vi "sub-Language buffer.vi"(7 "operation":enum16{"clear", "add", "get"}(ring), 10 "str":string, 11 "ID":u32 format="%04x") -> (2 "str out":string, 3 "ID out":u32)   [LabVIEW 2011]
panel:
  out "allid":u32[](array[numeric]) format="%04x"
  out "all":string[](array[string])
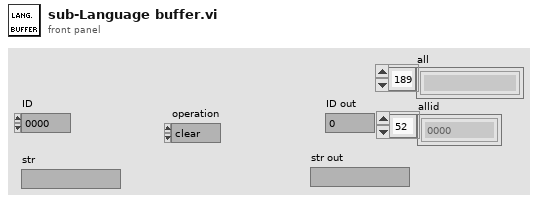
[diagram p1: front panel]
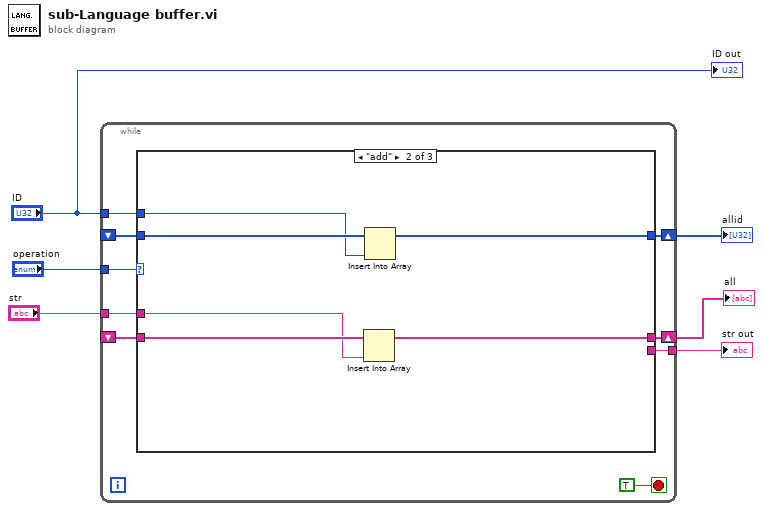
[diagram p0: block diagram]
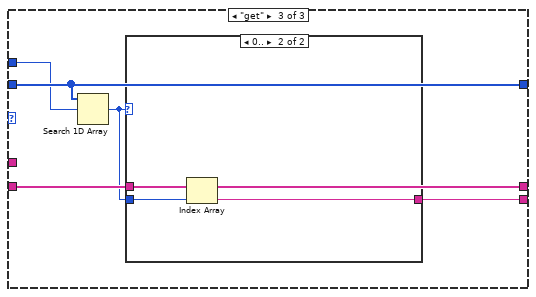
[diagram p3: hidden frame]
diagram:
  n1 = while {
    tunnel: "operation" -> [w14]
    tunnel: "ID" -> [w13]
    tunnel: "str" -> [w12]
    shift-right: [w9] -> w1
    shift-left: _ -> [w11]
    shift-right: [w8] -> w2
    shift-left: _ -> [w10]
    tunnel: [w7] -> w3
    stop <- TRUE stop-if-true
    n2 = case shown="\"add\"" w14 {
      tunnel: w13 -> [_ w20 w25]
      tunnel: w12 -> [_ w17 _]
      tunnel: w11 -> [_ w21 w26]
      tunnel: w10 -> [_ w18 w24]
      tunnel: [_ w19 w26] -> w9
      tunnel: [_ w16 w24] -> w8
      tunnel: [_ _ w22] -> w7
      frame "clear" {
      }
      frame "add" {
        n3 = Insert Into Array(array=w18, new element=w17) -> (w16:string[])  [unwired: 1 in]
        n4 = Insert Into Array(array=w21, new element=w20) -> (w19:u32[])  [unwired: 1 in]
      }
      frame "get" {
        n5 = Search 1D Array(1D array=w26, element=w25) -> (index of element=w23:i32)  [unwired: 1 in]
        n6 = case shown="0.." w23 {
          tunnel: w24 -> [_ w29]
          tunnel: w23 -> [_ w28]
          tunnel: [_ w27] -> w22
          frame -1, Default {
          }
          frame 0.. {
            n7 = Index Array(array=w29, index=w28) -> (element=w27:string)
          }
        }
      }
    }
  }
  "str out" <- w3
  "all" <- w2
  "allid" <- w1
  "ID out" <- "ID"
